vi "Add Waveform Section.vi"(8 "error in (no error)":errorcluster, 11 "Section Ptr":T1 format="%.0x") -> (0 "error out":errorcluster, 3 "Injector Section ptr":T1=18446744073709551615 format="%.0x")   [LabVIEW 2019, in "Fuel Injector Analysis Addon System Explorer.lvlib"]
uses:
  Fuel Injector Analysis Addon System Explorer.lvlib
  <vilib>/NI VeriStand/Custom Device API/Custom Device Item Ref.ctl
  <vilib>/NI VeriStand/Custom Device API/Custom Device Waveform.ctl
  <vilib>/NI VeriStand/Custom Device API/Custom Device Waveform DataType.ctl
  Addon Shared/SubVIs/Constants.vi
  <vilib>/NI VeriStand/Custom Device API/Custom Device API.lvlib
  Addon Shared/Fuel Injector Analysis Addon Shared.lvlib
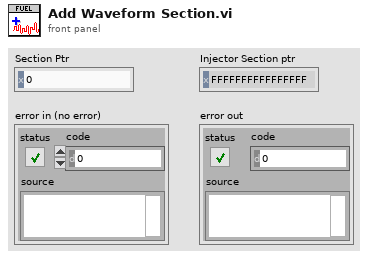
[diagram p1: front panel]
types:
  T1 = typedef "Custom Device API.lvlib/Custom Device Item Ref.ctl" = u64
  T2 = typedef "Custom Device API.lvlib/Custom Device Waveform.ctl" = cluster{"Data Type":T3, "Units":string}
  T3 = typedef "Custom Device API.lvlib/Custom Device Waveform DataType.ctl" = enum16{"Double", "Complex Double"}
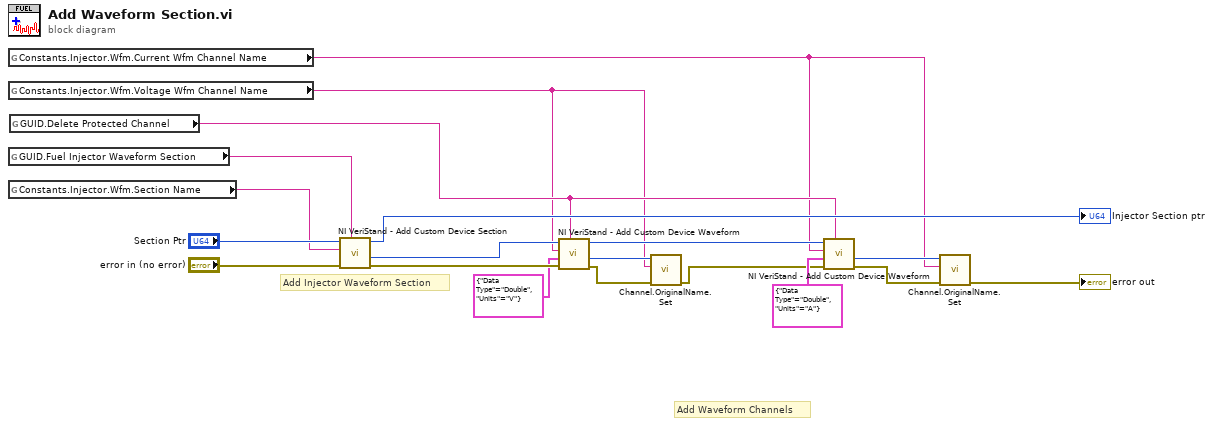
[diagram p0: block diagram]
diagram:
  # "Add Waveform Channels"
  # "Add Injector Waveform Section"
  n1 = global read "Constants.vi" "Constants.Injector.Wfm.Current Wfm Channel Name"() -> (w1:string)
  n2 = global read "Constants.vi" "Constants.Injector.Wfm.Voltage Wfm Channel Name"() -> (w5:string)
  n3 = global read "Constants.vi" "GUID.Fuel Injector Waveform Section"() -> (w17:string)
  n4 = global read "Constants.vi" "Constants.Injector.Wfm.Section Name"() -> (w15:string)
  n5 = global read "Constants.vi" "GUID.Delete Protected Channel"() -> (w10:string)
  n6 = call <vilib>:"NI VeriStand - Add Custom Device Section.vi"("GUID (Default Section)"=w17, "error in (no error)"="error in (no error)", "Section Name"=w15, "Parent Ref in"="Section Ptr") -> ("error out"=w14:errorcluster, "Section Ptr"=w18:T1, "Parent Ref out"=→"Injector Section ptr":T1)  [unwired: 4 in, 1 out]
  n7 = call <vilib>:"NI VeriStand - Add Custom Device Waveform.vi"("GUID (Default Waveform)"=w10, "error in (no error)"=w14, "Waveform"=T2 {"Data Type"=enum."Double", "Units"="V"}, "Waveform Name"=w5, "Parent Ref in"=w18) -> ("error out"=w9:errorcluster, "Waveform Ref"=w7:T1, "Parent Ref out"=w6:T1)  [unwired: 3 in, 1 out]
  n8 = call "Channel.OriginalName.Set.vi"("error in (no error)"=w9, "Constants.Channel Name"=w5, "Ref"=w7) -> ("error out"=w8:errorcluster)  [unwired: 7 in, 1 out]
  n9 = call <vilib>:"NI VeriStand - Add Custom Device Waveform.vi"("GUID (Default Waveform)"=w10, "error in (no error)"=w8, "Waveform"=T2 {"Data Type"=enum."Double", "Units"="A"}, "Waveform Name"=w1, "Parent Ref in"=w6) -> ("error out"=w4:errorcluster, "Waveform Ref"=w3:T1)  [unwired: 3 in, 2 out]
  n10 = call "Channel.OriginalName.Set.vi"("error in (no error)"=w4, "Constants.Channel Name"=w1, "Ref"=w3) -> ("error out"=→"error out":errorcluster)  [unwired: 7 in, 1 out]
